vi "dash_data_fg.vi"(1 "Input":bool=TRUE, 2 "DB DataType":T2, 3 "Menu (Get)":T3) -> (0 "Output":T1)   [LabVIEW 2011]
uses:
  fg_typedef.ctl
  DB DataType Custom.ctl
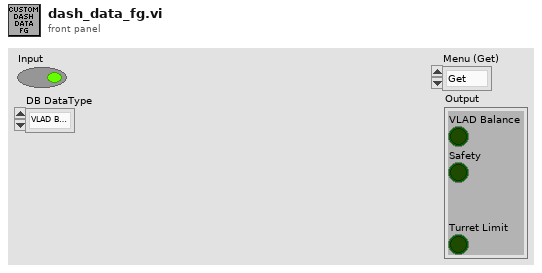
[diagram p1: front panel]
types:
  T1 = cluster{"VLAD Balance":bool, "Safety":bool, "Turret Limit":bool}
  T2 = typedef "DB DataType Custom.ctl" = enum16{"VLAD Balanced", "Turret Safety", "Turret Limit"}
  T3 = typedef "fg_typedef.ctl" = enum16{"Get", "Set"}
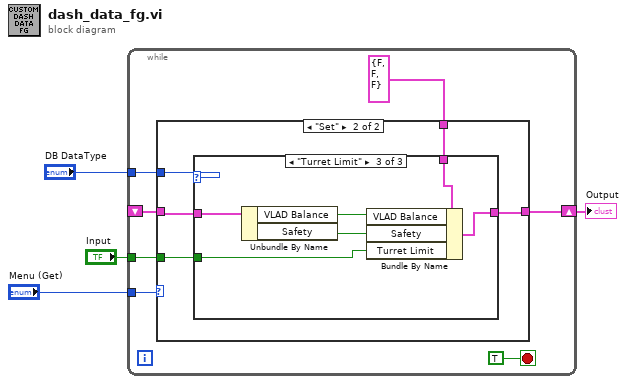
[diagram p0: block diagram]
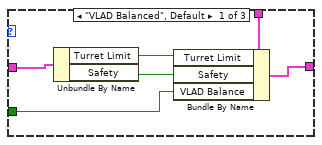
[diagram p3: hidden frame]
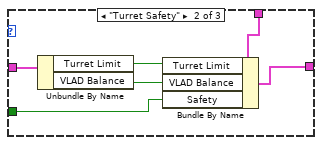
[diagram p4: hidden frame]
diagram:
  n1 = while {
    tunnel: "Menu (Get)" -> [w10]
    shift-right: [w7] -> w1
    shift-left: _ -> [w8]
    tunnel: "DB DataType" -> [w6]
    tunnel: "Input" -> [w5]
    stop <- TRUE stop-if-true
    n2 = case shown="\"Set\"" w10 {
      tunnel: T1 {"VLAD Balance"=FALSE, "Safety"=FALSE, "Turret Limit"=FALSE} ("Bools") -> [_ w16]
      tunnel: w8 -> [w12 w13]
      tunnel: [w12 w14] -> w7
      tunnel: w6 -> [_ w17]
      tunnel: w5 -> [_ w15]
      frame "Get", Default {
      }
      frame "Set" {
        n3 = case shown="\"Turret Limit\"" w17 {
          tunnel: w16 -> [w20 w26 w31]
          tunnel: w15 -> [w21 w24 w30]
          tunnel: [w19 w27 w32] -> w14
          tunnel: w13 -> [w22 w25 w33]
          frame "VLAD Balanced", Default {
            n4 = Unbundle By Name(w22) -> ("Turret Limit"=w18:bool, "Safety"=w23:bool)
            n5 = Bundle By Name(cluster=w20, "Turret Limit"=w18, "Safety"=w23, "VLAD Balance"=w21) -> (w19:T1)
          }
          frame "Turret Safety" {
            n6 = Unbundle By Name(w25) -> ("Turret Limit"=w28:bool, "VLAD Balance"=w29:bool)
            n7 = Bundle By Name(cluster=w26, "Turret Limit"=w28, "VLAD Balance"=w29, "Safety"=w24) -> (w27:T1)
          }
          frame "Turret Limit" {
            n8 = Unbundle By Name(w33) -> ("VLAD Balance"=w35:bool, "Safety"=w34:bool)
            n9 = Bundle By Name(cluster=w31, "VLAD Balance"=w35, "Safety"=w34, "Turret Limit"=w30) -> (w32:T1)
          }
        }
      }
    }
  }
  "Output" <- w1
